vi "CAN Get Value.vi"(7 "BufferLength":u32, 8 "error in (no error)":errorcluster, 9 "Buffer":u32, 10 "Parameter":u8, 11 "Channel":u16) -> (0 "error out":errorcluster, 1 "Buffer out":u32, 3 "function return":u32)   [LabVIEW 2017, in "PCANBasic_eX.lvlib"]
doc: "TPCANStatus __stdcall CAN_GetValue(\n TPCANHandle Channel, \n TPCANParameter Parameter, \n void* Buffer, \n DWORD BufferLength);"
uses:
  PCANBasic_eX.lvlib
  PCANBasic.dll
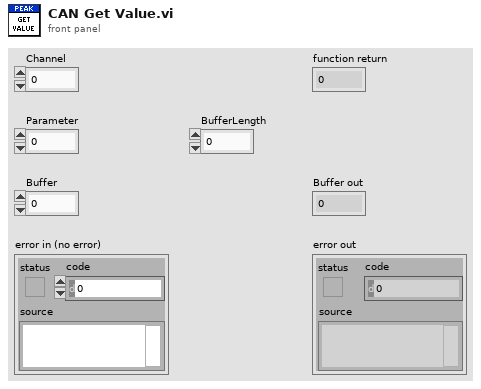
[diagram p1: front panel]
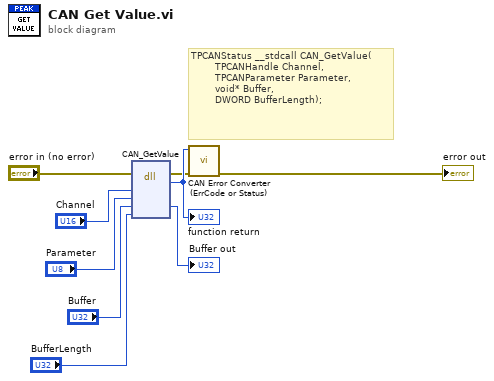
[diagram p0: block diagram]
diagram:
  # "TPCANStatus __stdcall CAN_GetValue(\n        TPCANHandle Channel, \n        TPCANParameter Parameter,  \n        void* Buffer, \n        DWORD BufferLength);"
  n1 = dll-call lib="PCANBasic.*" fn="CAN_GetValue"(error in="error in (no error)", "Channel"="Channel", "Parameter"="Parameter", "Buffer"="Buffer", "BufferLength"="BufferLength") -> (error out=w2:errorcluster, w9:u32, "Buffer"=→"Buffer out":u32)  [unwired: 5 in, 1 out]
  "function return" <- w9
  n2 = call "CAN Error Converter (ErrCode or Status).vi"("error in (no error)"=w2, "error code"=w9) -> ("error out"=→"error out":errorcluster)  [unwired: 9 in]
